vi "RT Loop - System Health and FPGA Monitoring.vi"(10 "FPGA VI Reference (Old)":T1, 11 "Message Queue":refnum<queue>) -> ()   [LabVIEW 2013]
uses:
  controls/FPGA VI Reference.ctl
  support/Message Queue/Message Cluster.ctl
  controls/FPGA State.ctl
  controls/Raw Values.ctl
  Globals/Global - Configuration Options.vi
  <vilib>/nisyscfg/Close (System).vi
  Globals/Global - All RT Loop Stop.vi
  <vilib>/Utility/error.llb/Error Cluster From Error Code.vi
  <vilib>/rvi/errors/niLvFpgaAdjustHostInterfaceError.vi
  <vilib>/rvi/interface/nirviReadWriteControl/nirviReadWriteControl.xnode
  FPGA Bitfiles/crio-FPGA-contro_FPGATarget_FPGAMain_4HKUk4gb9wY.lvbitx
  <vilib>/NI_Real-Time Target Support.lvlib
  <vilib>/nisyscfg/nisyscfg.lvlib
  <resource>/objmgr/nisysapi.rc
  NiFpgaLv.dll
  support/Message Queue/Message Queue.lvlib
panel:
  in  "FPGA VI Reference":refnum<k20>
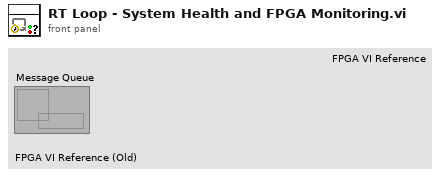
[diagram p1: front panel]
types:
  T1 = typedef "FPGA VI Reference.ctl" = refnum<k20>
  T2 = typedef "FPGA State.ctl" = enum16{"Safe State", "Manual", "Control (PID)"}
  T3 = typedef "Raw Values.ctl" = cluster{"Channel 0":fxp<+/-,20,7>, "Channel 1":fxp<+/-,20,7>, "Channel 2":fxp<+/-,20,7>, "Channel 3":fxp<+/-,20,14>}
  T4 = typedef "NI_Real-Time Target Support.lvlib/RT CPU Load.ctl" = cluster{"Total (%)":dbl, "Time Critical (%)":dbl, "Timed Structures (%)":dbl, "High (%)":dbl, "Above Normal (%)":dbl, "Normal (%)":dbl, "Background (%)":dbl, "Idle (%)":dbl, "ISR (%)":dbl}
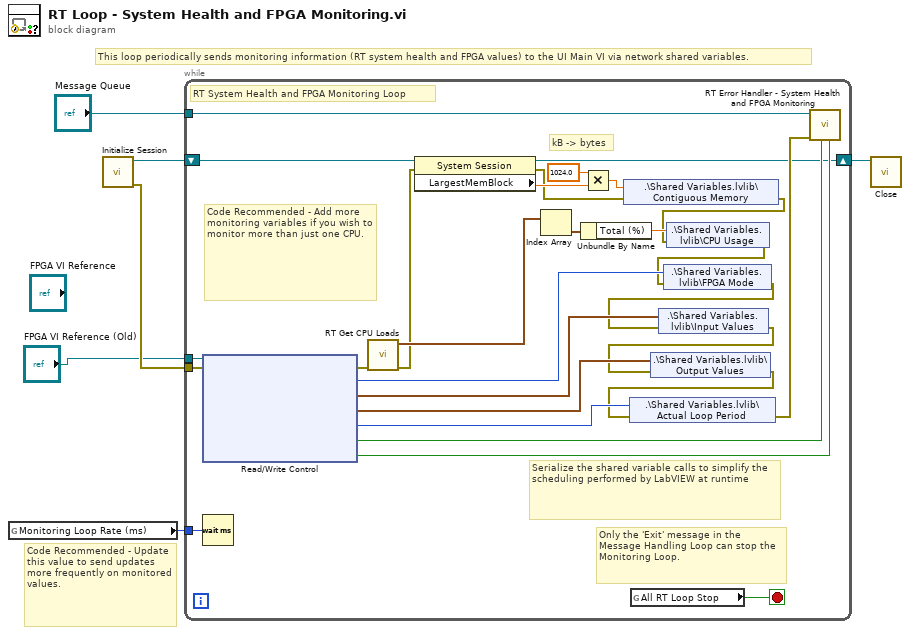
[diagram p0: block diagram]
diagram:
  # "Code Recommended - Update this value to send updates more frequently on monitored values."
  # "This loop periodically sends monitoring information (RT system health and FPGA values) to the UI Main VI via network shared variables."
  n1 = global read "Global - Configuration Options.vi" "Monitoring Loop Rate (ms)"() -> (w5:u32)
  n2 = call <vilib>:"Initialize Session.vi"() -> ("error out"=w2:errorcluster, "session out"=w4:refnum<k21>)  [unwired: 10 in]
  n3 = while {
    tunnel: "Message Queue" -> [w25]
    tunnel: "FPGA VI Reference (Old)" -> [w28]
    tunnel: w5 -> [w24]
    shift-right: [w10] -> w3
    shift-left: w4 -> [w14]
    tunnel: w2 -> [w7]
    stop <- w26 stop-if-true
    # "kB -> bytes"
    # "Serialize the shared variable calls to simplify the scheduling performed by LabVIEW at runtime"
    # "Code Recommended - Add more monitoring variables if you wish to monitor more than just one CPU."
    # "Only the 'Exit' message in the  Message Handling Loop can stop the Monitoring Loop."
    # "RT System Health and FPGA Monitoring Loop"
    n4 = xnode "Read/Write Control"("FPGA VI Reference In"=w28, "error in"=w7) -> ("error out"=w21:errorcluster, "Current FPGA State"=w29:T2, "Input Values"=w30:T3, "Output Values"=w31:T3, "Actual Loop Period (ticks)"=w27:u32, "Input Error"=w23:bool, "Output Error"=w22:bool)  [unwired: 1 out]
    n5 = Wait (ms)(milliseconds to wait=w24) -> ()  [unwired: 1 out]
    n6 = call <vilib>:"RT Get CPU Loads.vi"("error in (no error)"=w21) -> ("error out"=w12:errorcluster, "CPU loads"=w34:T4[])  [unwired: 9 in]
    n7 = property class="System Session"(reference=w14, error in=w12) -> (reference out=w10:refnum<k21>, error out=w11:errorcluster, "LargestMemBlock"=w13:dbl)
    n8 = Index Array(array=w34) -> (element=w33:T4)  [unwired: 1 in]
    n9 = Unbundle By Name(w33) -> ("Total (%)"=w32:dbl)
    n10 = Multiply(x=1024.0, y=w13) -> (x*y=w9:dbl)
    n11 = shared-variable ".\\Shared Variables.lvlib\\Contiguous Memory"(w9, error in=w11) -> (error out=w16:errorcluster)
    n12 = global read "Global - All RT Loop Stop.vi" "All RT Loop Stop"() -> (w26:bool)
    n13 = shared-variable ".\\Shared Variables.lvlib\\CPU Usage"(w32, error in=w16) -> (error out=w15:errorcluster)
    n14 = shared-variable ".\\Shared Variables.lvlib\\FPGA Mode"(w29, error in=w15) -> (error out=w20:errorcluster)
    n15 = shared-variable ".\\Shared Variables.lvlib\\Input Values"(w30, error in=w20) -> (error out=w19:errorcluster)
    n16 = shared-variable ".\\Shared Variables.lvlib\\Output Values"(w31, error in=w19) -> (error out=w18:errorcluster)
    n17 = shared-variable ".\\Shared Variables.lvlib\\Actual Loop Period"(w27, error in=w18) -> (error out=w17:errorcluster)
    n18 = call "RT Error Handler - System Health and FPGA Monitoring.vi"("Output Error (FPGA)"=w22, "Input Error (FPGA)"=w23, "error in (no error)"=w17, "Message Queue"=w25) -> ()  [unwired: 7 in, 1 out]
  }
  n19 = call-poly <vilib>:"Close.vi"("session in"=w3) -> ()  [unwired: 10 in, 1 out]
